vi "Model Select.vi"() -> (2 "Next action":bool)   [LabVIEW 2015]
uses:
  Feature list/Control PB/Next_.ctl
  Galobal variable_TI.vi
panel:
  in  "Next":T1
  in  "Exit":bool
  in  "Model":u16(ring) items=["Select The Model", "38400-72R00", "38400-72R20", "38400-72R10"]
  out "Array":string[](array[string])
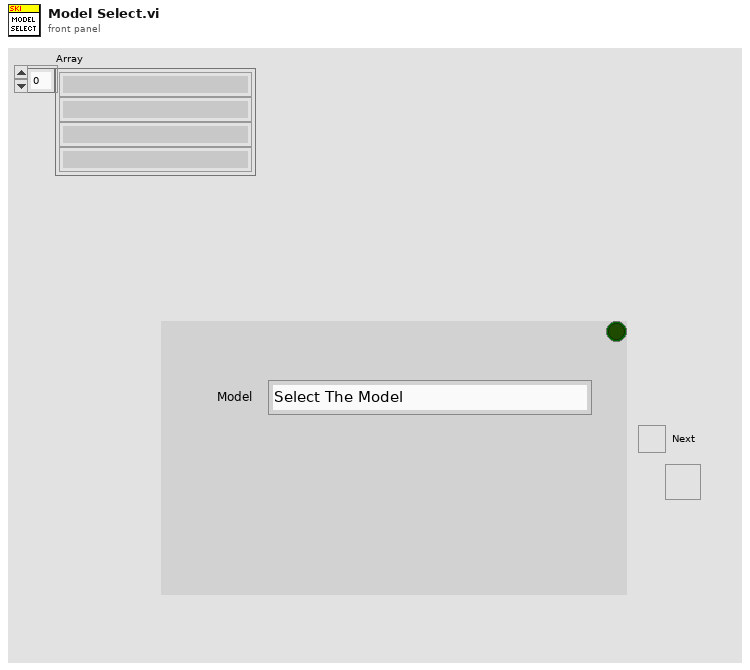
[diagram p1: front panel]
types:
  T1 = typedef "Next_.ctl" = bool
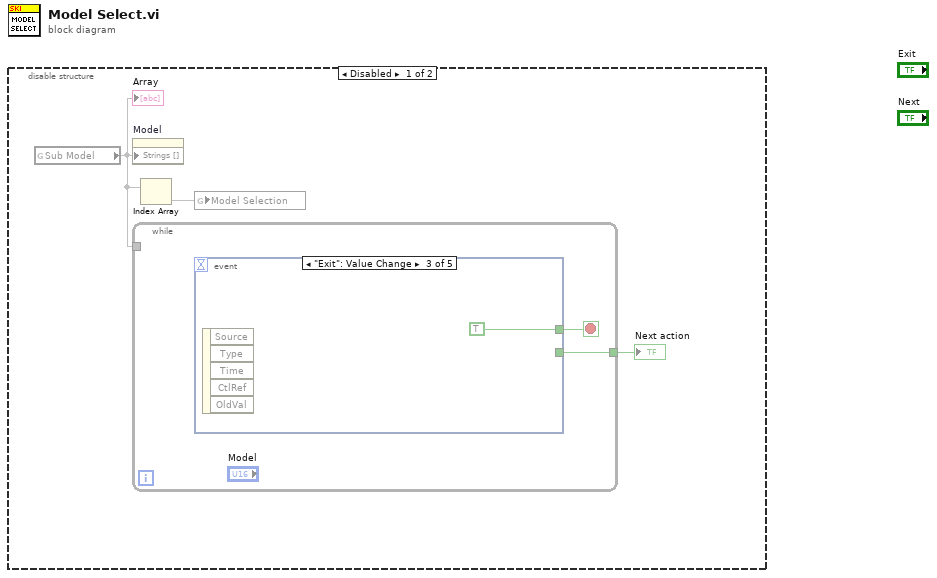
[diagram p0: block diagram]
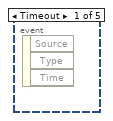
[diagram p2: hidden frame]
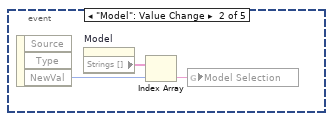
[diagram p3: hidden frame]
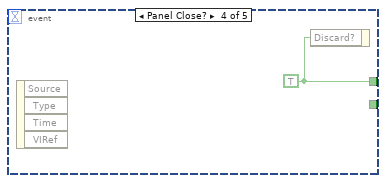
[diagram p4: hidden frame]
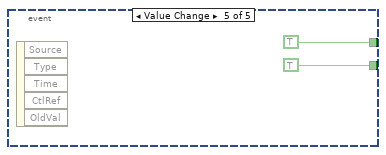
[diagram p5: hidden frame]
diagram:
  n1 = disable-structure shown="Disabled" {
    frame Disabled {
      n2 = global read "Galobal variable_TI.vi" "Sub Model"() -> (w1)
      "Array" <- w1
      n3 = property on="Model" class="Ring (strict)"("Strings []"=w1) -> ()  [unwired: 2 in, 2 out]
      n4 = while {
        tunnel: [w4] -> w3
        tunnel: w1 -> [_]
        stop <- w5 stop-if-true
        n5 = event shown="[2] \"Exit\": Value Change" {
          selector: _ -> [_ _ _ _ _]
          dyn-events: _ -> [_ _ _ _ _]
          timeout: _ -> [_ _ _ _ _]
          tunnel: [_ _ TRUE w10 TRUE] -> w5
          tunnel: [_ _ _ _ TRUE] -> w4
          event Timeout {
            n6 = event-data() -> ()  [unwired: 1 in, 3 out]
          }
          event "Model": Value Change {
            n7 = event-data() -> ("NewVal"=w7:u16)  [unwired: 1 in, 2 out]
            n8 = property on="Model" class="Ring (strict)"() -> ("Strings []"=w8:string[])  [unwired: 2 in, 2 out]
            n9 = Index Array(array=w8, index=w7) -> (element=w6:string)
            n10 = global write "Galobal variable_TI.vi" "Model Selection"(w6) -> ()
          }
          event "Exit": Value Change {
            n11 = event-data() -> ()  [unwired: 1 in, 5 out]
          }
          event Panel Close? {
            w10 = TRUE ("Discard?")
            n12 = event-data() -> ()  [unwired: 1 in, 4 out]
            n13 = event-data("Discard?"=w10) -> ()  [unwired: 1 in, 1 out]
          }
          event Value Change {
            n14 = event-data() -> ()  [unwired: 1 in, 5 out]
          }
        }
      }
      "Next action" <- w3
      n15 = Index Array(array=w1) -> (element=w2)  [unwired: 1 in]
      n16 = global write "Galobal variable_TI.vi" "Model Selection"(w2) -> ()
    }
    frame Enabled {
    }
  }
